vi "subMFD_FXP CodeGen.vi"() -> ()   [LabVIEW 2023]
uses:
  <vilib>/addons/Digital Filter Design/_Objects.llb/DFD Multirate Filter Obj.ctl
  <vilib>/addons/Digital Filter Design/_Objects.llb/DFD Multirate Mode.ctl
  <vilib>/addons/Digital Filter Design/_Objects.llb/DFD Coef Norm Type.ctl
  <vilib>/addons/Digital Filter Design/_Objects.llb/DFD Round-off Mode.ctl
  <vilib>/addons/Digital Filter Design/_Objects.llb/DFD FXP MRate Multiply Mode.ctl
  <vilib>/Utility/error.llb/ErrWarn.ctl
  <vilib>/addons/Digital Filter Design/NI_DigFilterLicensed.lvlib
panel:
  in  "View Option":enum32{"proj", "code"}(radio)
  out "Code Example":u16(ring)
  out "Message":string="Specify the Code Generation Settings and click the Generate Code button to generate LabVIEW FPGA code from the fixed-point multirate filter."
  out "Maximum Input Fs@40 MHz FPGA Clock":string
  out "error":T1=TRUE
  in  "# Channels":i32=1
  in  "Filter Name":string="MyMRateFilter"
  in  "Destination Folder":path
  out "Successful Design?":bool
  out "multirate filter out":T2={"mMRate_Structure"=enum."FIR", "mMRate_Mode"=0, "mMRate_Factor"=-1, "mMRate_FIRParams"={"mMRate_FIR_H"=[], "mMRate_FIR_IsNyquist?"=FALSE, "mMRate_FIR_IsSymmetric?"=FALSE}, "mMRate_CICParams"={"mMRate_CIC_#Stage"=0, "mMRate_CIC_Lag"=1, "mMRate_CIC_Type"=enum."Lowpass"}, "mMRate_Order"=0, "mMRate_Version"="2.0", "mMRate_Comments"="", "mMRate_RationalFactor"={"mMRate_L"=-1, "mMRate_M"=-1}, "mMRate_Fs"=1.0, "mMRate_Quantized?"=FALSE, "mMRate_QFilterGain"=1.0, "mMRate_CoefWl"=16, "mMRate_Scaling"={"mMRate_ScaleByPowerOf2?"=FALSE, "mMRate_ScaleType"=enum."No Norm"}, "mMRate_InputWl"=16, "mMRate_OutputWl"=16, "mMRate_OutputMode"=enum."Truncation", "mMRate_MultMode"=enum."Truncated", "mMRate_BitPruning"=FALSE, "mMRate_GainWl"=16, "mMRate_OutputFwl"=0, "mMRate_SumIwl"=0, "mMRate_InputIwl "=16, "mMRate_SumWl"=32, "mMRate_CoefIwl"=0} {"mMRate_SumWl" min=1 max=32 step=1; "mMRate_InputIwl" min=1 max=32 step=1; "mMRate_GainWl" min=1 max=32 step=1; "mMRate_OutputWl" min=1 max=32 step=1; "mMRate_InputWl" min=1 max=32 step=1; "mMRate_CoefWl" min=1 max=32 step=1; "mMRate_Mode" items=["Default"=-1, "No Rate Change"=0, "Interpolation"=1, "Decimation"=2, "Interpolated"=3, "Rational"=4]}
  in  "multirate filter in":T2={"mMRate_Structure"=enum."FIR", "mMRate_Mode"=0, "mMRate_Factor"=-1, "mMRate_FIRParams"={"mMRate_FIR_H"=[], "mMRate_FIR_IsNyquist?"=FALSE, "mMRate_FIR_IsSymmetric?"=FALSE}, "mMRate_CICParams"={"mMRate_CIC_#Stage"=0, "mMRate_CIC_Lag"=1, "mMRate_CIC_Type"=enum."Lowpass"}, "mMRate_Order"=0, "mMRate_Version"="2.0", "mMRate_Comments"="", "mMRate_RationalFactor"={"mMRate_L"=-1, "mMRate_M"=-1}, "mMRate_Fs"=1.0, "mMRate_Quantized?"=FALSE, "mMRate_QFilterGain"=1.0, "mMRate_CoefWl"=16, "mMRate_Scaling"={"mMRate_ScaleByPowerOf2?"=FALSE, "mMRate_ScaleType"=enum."No Norm"}, "mMRate_InputWl"=16, "mMRate_OutputWl"=16, "mMRate_OutputMode"=enum."Truncation", "mMRate_MultMode"=enum."Truncated", "mMRate_BitPruning"=FALSE, "mMRate_GainWl"=16, "mMRate_OutputFwl"=0, "mMRate_SumIwl"=0, "mMRate_InputIwl "=16, "mMRate_SumWl"=32, "mMRate_CoefIwl"=0} {"mMRate_SumWl" min=1 max=32 step=1; "mMRate_InputIwl" min=1 max=32 step=1; "mMRate_GainWl" min=1 max=32 step=1; "mMRate_OutputWl" min=1 max=32 step=1; "mMRate_InputWl" min=1 max=32 step=1; "mMRate_CoefWl" min=1 max=32 step=1; "mMRate_Mode" items=["Default"=-1, "No Rate Change"=0, "Interpolation"=1, "Decimation"=2, "Interpolated"=3, "Rational"=4]}
  in  "Generate Code":bool
  out "OK":bool
  in  "stop":bool
  # "Code Example"
  # "Code Generation Settings"
  # "Code Generation Feedback"
  # "View Option"
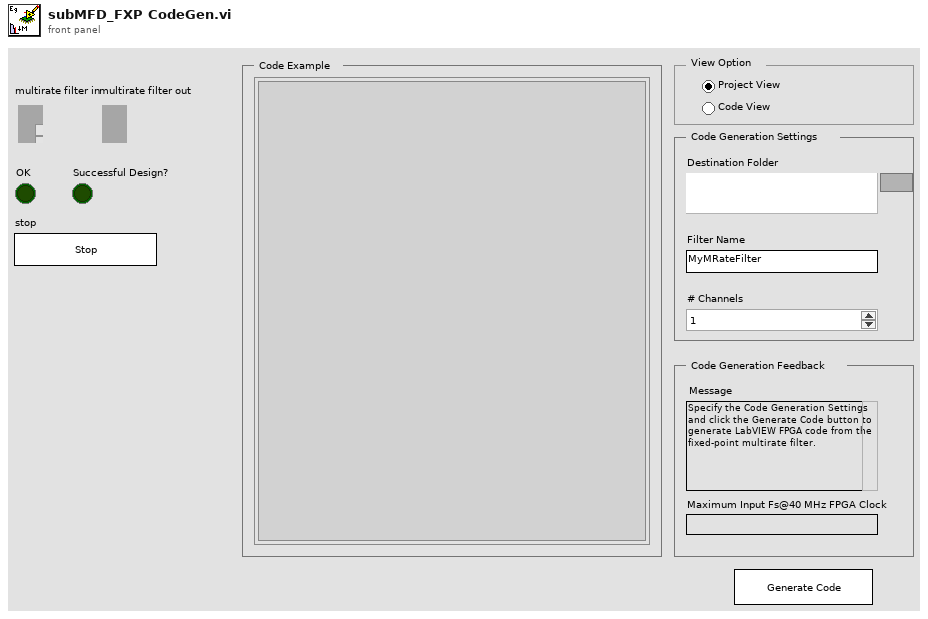
[diagram p1: front panel]
types:
  T1 = typedef "ErrWarn.ctl" = bool
  T2 = typedef "NI_DigFilterLicensed.lvlib/DFD Multirate Filter Obj.ctl" = cluster{"mMRate_Structure":enum16{"CIC", "FIR", "IIR", "Lattice"}, "mMRate_Mode":T3, "mMRate_Factor":i32, "mMRate_FIRParams":cluster{"mMRate_FIR_H":dbl[], "mMRate_FIR_IsNyquist?":bool, "mMRate_FIR_IsSymmetric?":bool}, "mMRate_CICParams":cluster{"mMRate_CIC_#Stage":i32, "mMRate_CIC_Lag":i32, "mMRate_CIC_Type":enum16{"Lowpass", "Highpass"}}, "mMRate_Order":i32, "mMRate_Version":string, "mMRate_Comments":string, "mMRate_RationalFactor":cluster{"mMRate_L":i32, "mMRate_M":i32}, "mMRate_Fs":dbl, "mMRate_Quantized?":bool, "mMRate_QFilterGain":dbl, "mMRate_CoefWl":i16, "mMRate_Scaling":cluster{"mMRate_ScaleByPowerOf2?":bool, "mMRate_ScaleType":T4}, "mMRate_InputWl":i16, "mMRate_OutputWl":i16, "mMRate_OutputMode":T5, "mMRate_MultMode":T6, "mMRate_BitPruning":bool, "mMRate_GainWl":i16, "mMRate_OutputFwl":i16, "mMRate_SumIwl":i16, "mMRate_InputIwl ":i16, "mMRate_SumWl":i16, "mMRate_CoefIwl":i16}
  T3 = typedef "NI_DigFilterLicensed.lvlib/DFD Multirate Mode.ctl" = i16
  T4 = typedef "NI_DigFilterLicensed.lvlib/DFD Coef Norm Type.ctl" = enum16{"No Norm", "Time Domain 1-Norm", "Time Domain 2-Norm", "Time Domain Inf-Norm"}
  T5 = typedef "NI_DigFilterLicensed.lvlib/DFD Round-off Mode.ctl" = enum16{"Nearest", "Truncation"}
  T6 = typedef "NI_DigFilterLicensed.lvlib/DFD FXP MRate Multiply Mode.ctl" = enum16{"Truncated", "Full"}
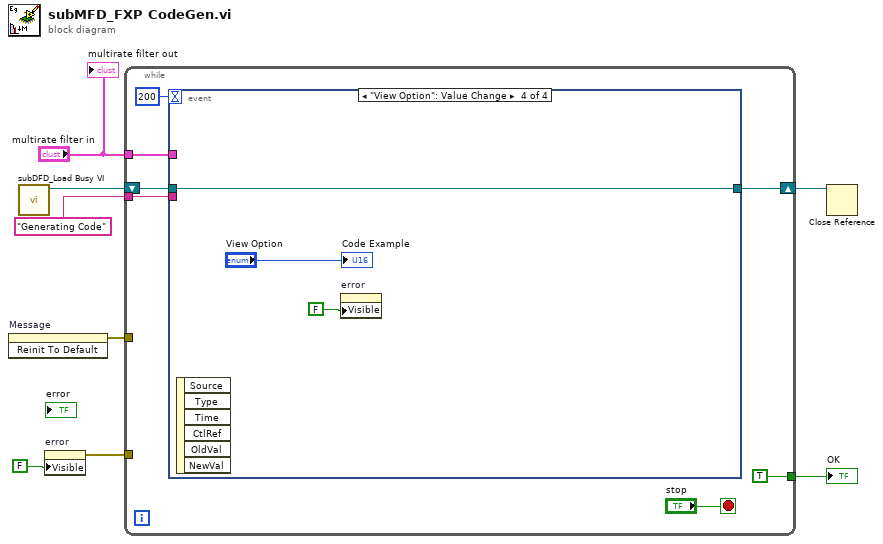
[diagram p0: block diagram]
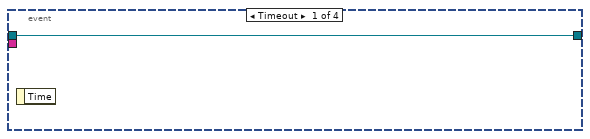
[diagram p2: hidden frame]
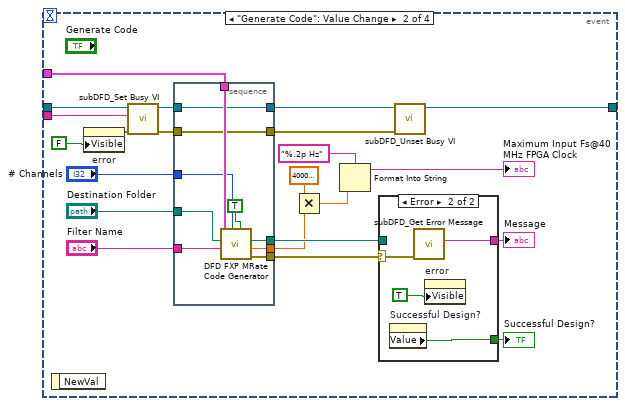
[diagram p3: hidden frame]
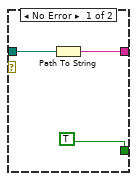
[diagram p4: hidden frame]
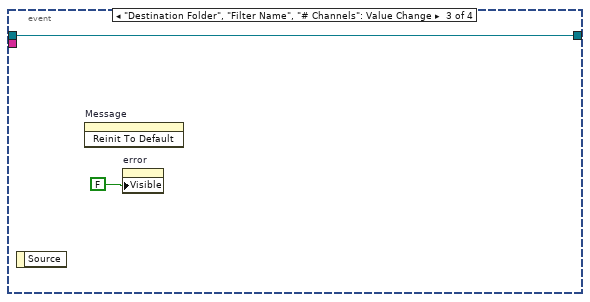
[diagram p5: hidden frame]
diagram:
  n1 = invoke on="Message" class="Str" method="Reinit To Default"() -> (error out=w3:errorcluster)  [unwired: 3 in, 2 out]
  n2 = call <vilib>:"subDFD_Load Busy VI.vi"() -> ("Busy vi reference"=w2:refnum<vi>)  [unwired: 11 out]
  n3 = property on="error" class="Bool"("Visible"=FALSE) -> (error out=w4:errorcluster)  [unwired: 2 in, 1 out]
  n4 = while {
    tunnel: [TRUE] -> w8
    tunnel: "multirate filter in" -> [w12]
    shift-right: [w10] -> w6
    shift-left: w2 -> [w11]
    tunnel: w4 -> [_]
    tunnel: w3 -> [_]
    tunnel: "Generating Code" ("control name") -> [w9]
    stop <- "stop" stop-if-true
    n5 = event shown="[3] \"View Option\": Value Change" {
      selector: _ -> [_ _ _ _]
      dyn-events: _ -> [_ _ _ _]
      timeout: 200 -> [_ _ _ _]
      tunnel: w12 -> [_ w38 _ _]
      tunnel: w11 -> [w16 w32 w57 w60]
      tunnel: [w16 w33 w57 w60] -> w10
      tunnel: w9 -> [_ w17 _ _]
      event Timeout {
        n6 = event-data() -> ()  [unwired: 2 out]
      }
      event "Generate Code": Value Change {
        n7 = event-data() -> ()  [unwired: 2 out]
        n8 = property on="error" class="Bool"("Visible"=FALSE) -> (error out=w18:errorcluster)  [unwired: 2 in, 1 out]
        n9 = call <vilib>:"subDFD_Set Busy VI.vi"("error in (no error)"=w18, "busy task"=w17, "Busy vi reference"=w32) -> ("error out"=w25:errorcluster, "dup Busy vi reference"=w26:refnum<vi>)  [unwired: 7 out]
        n10 = stacked-sequence {
          tunnel: w38 -> [w48]
          tunnel: "Filter Name" -> [w47]
          tunnel: "Destination Folder" -> [w46]
          tunnel: "# Channels" -> [w45]
          tunnel: [w44] -> w34
          tunnel: [w43] -> w31
          tunnel: [w42] -> w30
          tunnel: [w40] -> w23
          tunnel: w26 -> [w40]
          tunnel: w25 -> [w39]
          tunnel: [w39] -> w24
          frame #0 {
            n11 = call <vilib>:"DFD FXP MRate Code Generator.vi"("open project? (F)"=TRUE ("open FP? (F)"), "# channels"=w45, "filter name"=w47, "destination folder"=w46, "multirate filter"=w48) -> ("error out"=w44:errorcluster, "sampling frequency/FPGA clock"=w42:dbl, "lvproj path"=w43:path)  [unwired: 2 in, 2 out]
          }
        }
        n12 = Multiply(x=40000000.0, y=w30) -> (x*y=w21:dbl)
        n13 = Format Into String(format string="%.2p Hz", w21) -> (resulting string=→"Maximum Input Fs@40 MHz FPGA Clock":string)  [unwired: 2 in, 1 out]
        n14 = case shown="Error" w34 {
          selector: w34 -> [_ w55]
          tunnel: [w50 w54] -> w28
          tunnel: w31 -> [w51 _]
          tunnel: [TRUE ("Successful Design?") w52] -> w27
          frame No Error {
            n15 = Path To String(path=w51) -> (string=w50:string)
          }
          frame Error {
            n16 = property on="Successful Design?" class="Bool (strict)"() -> ("Value"=w52:bool)  [unwired: 2 in, 2 out]
            n17 = call <vilib>:"subDFD_Get Error Message.vi"("error in (no error)"=w55) -> ("Error Message"=w54:string)  [unwired: 10 out]
            n18 = property on="error" class="Bool"("Visible"=TRUE) -> ()  [unwired: 2 in, 2 out]
          }
        }
        "Successful Design?" <- w27
        "Message" <- w28
        n19 = call <vilib>:"subDFD_Unset Busy VI.vi"("error in (no error)"=w24, "Busy vi reference"=w23) -> ("dup Busy vi reference"=w33:refnum<vi>)  [unwired: 9 out]
      }
      event "Destination Folder", "Filter Name", "# Channels": Value Change {
        n20 = event-data() -> ()  [unwired: 2 out]
        n21 = invoke on="Message" class="Str" method="Reinit To Default"() -> ()  [unwired: 3 in, 3 out]
        n22 = property on="error" class="Bool"("Visible"=FALSE) -> ()  [unwired: 2 in, 2 out]
      }
      event "View Option": Value Change {
        n23 = event-data() -> ()  [unwired: 7 out]
        n24 = property on="error" class="Bool"("Visible"=FALSE) -> ()  [unwired: 2 in, 2 out]
        "Code Example" <- "View Option"
      }
    }
  }
  "OK" <- w8
  n25 = Close Reference(reference=w6) -> ()  [unwired: 1 in, 1 out]
  "multirate filter out" <- "multirate filter in"
